vi "servo_client.vi"() -> ()   [LabVIEW 2019]
doc: "演示连接TCP服务器、读取发送的数据并在图表上显示数据的方法。VI设计为TCP连接断开时停止。"
panel:
  out "字符串":string
  in  "Position":dbl(ring) items=["start"=0.0, "end"=180.0]
  out "错误输出":errorcluster
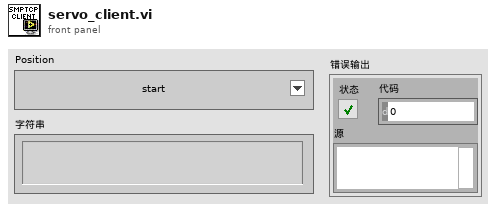
[diagram p1: front panel]
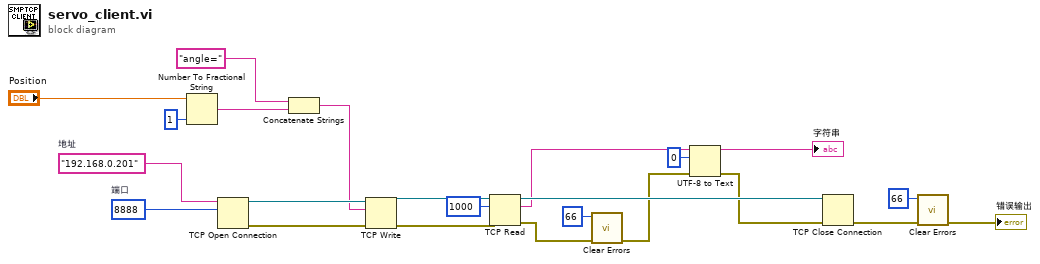
[diagram p0: block diagram]
diagram:
  w20 = u16 8888  # 端口
  w21 = "192.168.0.201"  # 地址
  n1 = Number To Fractional String(number="Position", precision (6)=i16 1 ("精度(6)")) -> (F-format string=w18:string)  [unwired: 2 in]
  n2 = TCP Open Connection(address=w21, remote port or service name=w20) -> (connection ID=w23:refnum<k5>, error out=w22:errorcluster)  [unwired: 3 in]
  n3 = Concatenate Strings("angle=" ("数据输入"), w18) -> (w17:string)
  n4 = TCP Write(connection ID=w23, data in=w17, error in (no error)=w22) -> (connection ID out=w14:refnum<k5>, error out=w13:errorcluster)  [unwired: 1 in, 1 out]
  n5 = TCP Read(connection ID=w14, bytes to read=1000 ("读取的字节"), error in (no error)=w13) -> (connection ID out=w12:refnum<k5>, data out=w10:string, error out=w2:errorcluster)  [unwired: 2 in]
  n6 = call <vilib>:"Clear Errors.vi"("error in (no error)"=w2, "specific error code to clear (0: all)"=66) -> ("error out"=w1:errorcluster)  [unwired: 4 in, 1 out]
  n7 = UTF-8 to Text(8:w1, 10:0 ("编码（系统默认=-1）"), 11:w10) -> (0:w9:errorcluster, 3:→"字符串":string)
  n8 = TCP Close Connection(connection ID=w12, error in (no error)=w9) -> (error out=w7:errorcluster)  [unwired: 1 in, 1 out]
  n9 = call <vilib>:"Clear Errors.vi"("error in (no error)"=w7, "specific error code to clear (0: all)"=66) -> ("error out"=→"错误输出":errorcluster)  [unwired: 4 in, 1 out]
